vi "Align Scanner.vi"(9 "New Scanner":T1, 11 "Known Scanners":T1[](array[typedef])) -> (0 "Aligned?":bool, 1 "Updated Scanner":T1, 2 "Best Scanner Index":i32, 3 "Max Overlap":i32)   [LabVIEW 2020]
uses:
  Scanner.ctl
  Vec3.ctl
  <vilib>/Utility/miscctls.llb/LVMapReplaceAction.ctl
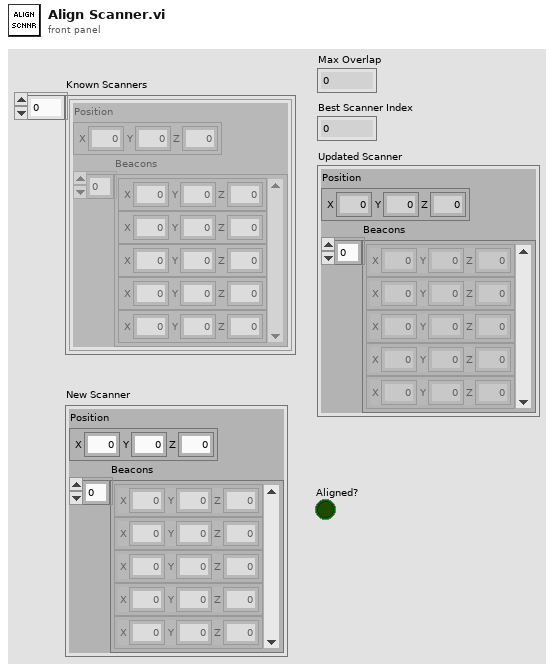
[diagram p1: front panel]
types:
  T1 = typedef "Scanner.ctl" = cluster{"Position":T2, "Beacons":T2[]}
  T2 = typedef "Vec3.ctl" = cluster{"X":dbl, "Y":dbl, "Z":dbl}
  T3 = typedef "NI_Matrix.lvlib/RealMatrix.ctl" = dbl[][]
  T4 = typedef "LVMapReplaceAction.ctl" = enum32{"Modify Entry only if found", "Add or Modify Entry", "Delete Entry"}
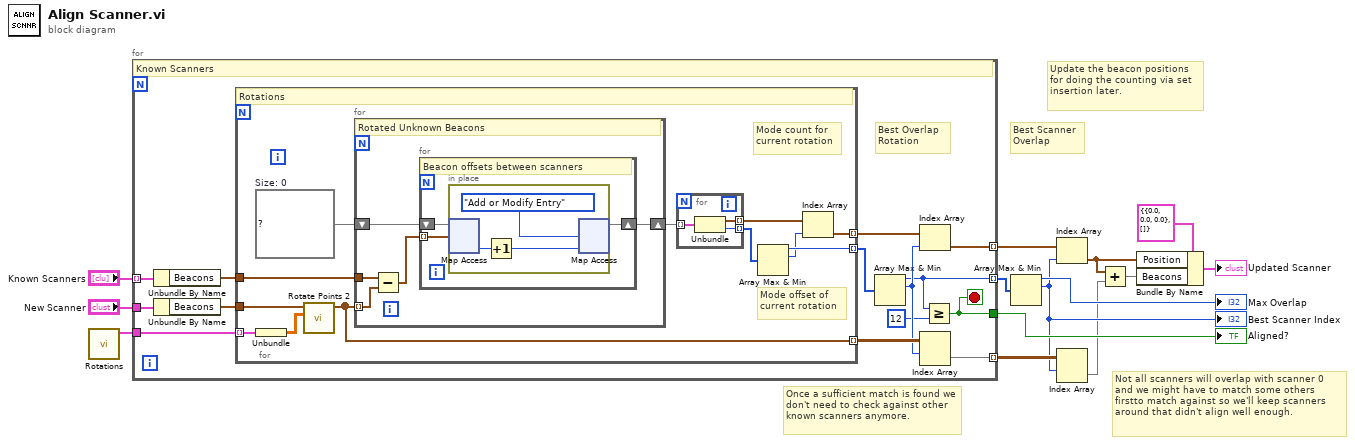
[diagram p0: block diagram]
diagram:
  # "Not all scanners will overlap with scanner 0 and we might have to match some others firstto match against so we'll keep scanners around that didn't align well enough."
  # "Update the beacon positions for doing the counting via set insertion later."
  # "Once a sufficient match is found we don't need to check against other known scanners anymore."
  # "Best Scanner Overlap"
  n1 = call "Rotations.vi"() -> ("Rotations"=w11:cluster{"Rotation":T3}[])  [unwired: 11 in]
  n2 = for {
    tunnel: "Known Scanners" -> [w28] mode=indexing
    tunnel: "New Scanner" -> [w26]
    tunnel: w11 -> [w24]
    tunnel: [w17] -> w9 mode=indexing
    tunnel: [w21] -> w7 mode=indexing
    tunnel: [w18] -> w6 mode=indexing
    tunnel: [w15] -> w14
    stop <- w15 stop-if-true
    # "Best Overlap Rotation"
    # "Known Scanners"
    n3 = Unbundle By Name(w28) -> ("Beacons"=w27:T2[])
    n4 = Unbundle By Name(w26) -> ("Beacons"=w25:T2[])
    n5 = for {
      tunnel: w27 -> [w38]
      tunnel: w25 -> [w40]
      tunnel: w24 -> [w39] mode=indexing
      tunnel: [w33] -> w23 mode=indexing
      tunnel: [w32] -> w20 mode=indexing
      tunnel: [w29] -> w22 mode=indexing
      w37 = map{T2, i32} {}  # Size: 0
      # "Mode offset of current rotation"
      # "Mode count for current rotation"
      # "Rotations"
      n6 = Unbundle(w39) -> ("Rotation"=w36:T3)
      n7 = call "Rotate Points 2.vi"("Rotation Matrix"=w36, "Positions"=w40) -> ("Rotated"=w32:T2[])  [unwired: 9 in]
      n8 = for {
        tunnel: w32 -> [w47] mode=indexing
        tunnel: w38 -> [w48]
        shift-right: [w44] -> w35
        shift-left: w37 -> [w46]
        # "Rotated Unknown Beacons"
        n9 = Subtract(x=w48, y=w47) -> (x-y=w45:T2[])
        n10 = for {
          shift-right: [w50] -> w44
          shift-left: w46 -> [w51]
          tunnel: w45 -> [w49] mode=indexing
          # "Beacon offsets between scanners"
          n11 = in-place {
            n12 = in-place-map #1(w51, w49) -> (w54:i32)  [unwired: 1 in, 1 out]
            n13 = Increment(x=w54) -> (x+1=w53:i32)
            n14 = in-place-map #1(w53, LVMapReplaceAction."Add or Modify Entry" ("action")) -> (w50:map{T2, i32})  [unwired: 2 out]
          }
        }
      }
      n15 = for {
        tunnel: w35 -> [w43] mode=indexing
        tunnel: [w42] -> w34 mode=indexing
        tunnel: [w41] -> w31 mode=indexing
        n16 = Unbundle(w43) -> ("Position"=w41:T2, w42:i32)
      }
      n17 = Array Max & Min(array=w34) -> (max value=w33:i32, max index (indices)=w30:i32)  [unwired: 2 out]
      n18 = Index Array(array=w31, index=w30) -> (element=w29:T2)
    }
    n19 = Array Max & Min(array=w23) -> (max value=w17:i32, max index (indices)=w19:i32)  [unwired: 2 out]
    n20 = Index Array(array=w22, index=w19) -> (element=w21:T2)
    n21 = Index Array(array=w20, index (row)=w19) -> (element=w18:T2[])  [unwired: 1 in]
    n22 = Greater Or Equal?(x=w17, y=12) -> (x >= y?=w15:bool)
  }
  "Aligned?" <- w14
  n23 = Array Max & Min(array=w9) -> (max value=→"Max Overlap":i32, max index (indices)=w5:i32)  [unwired: 2 out]
  "Best Scanner Index" <- w5
  n24 = Index Array(array=w7, index=w5) -> (element=w1:T2)
  n25 = Index Array(array=w6, index (row)=w5) -> (element=w3:T2[])  [unwired: 1 in]
  n26 = Add(x=w1, y=w3) -> (x+y=w2:T2[])
  n27 = Bundle By Name(cluster=T1 {"Position"={"X"=0.0, "Y"=0.0, "Z"=0.0}, "Beacons"=[]} ("Scanner"), "Position"=w1, "Beacons"=w2) -> (→"Updated Scanner":T1)
